vi "read station misc config.vi"(8 "error in":errorcluster, 10 "station idx":i32, 11 "configuration file path in":path) -> (0 "error out":errorcluster, 2 "misc station config":T1, 3 "configuration file path out":path)   [LabVIEW 2018]
uses:
  02.Type Def's/misc station config.ctl
  05.UserVI's/Lambda Power/power supply types.ctl
  05.UserVI's/file io/ini/type defs/ini file actions.ctl
  05.UserVI's/file io/ini/type defs/ini entry value.ctl
  05.UserVI's/file io/ini/type defs/ini entry types.ctl
  05.UserVI's/file io/ini/type defs/ini entry.ctl
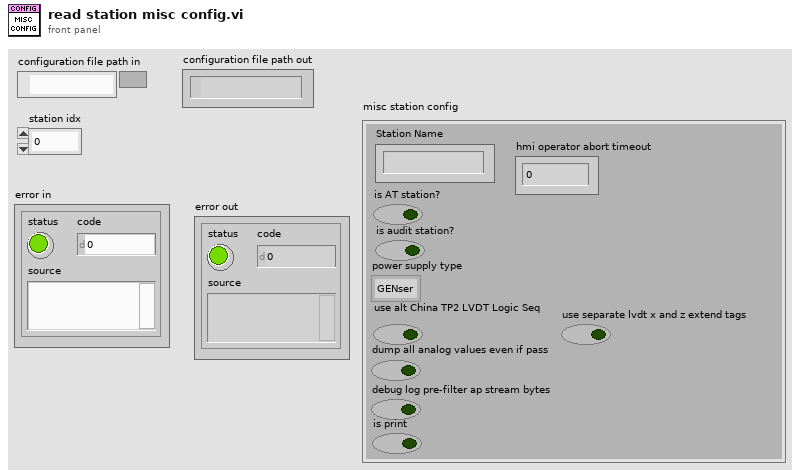
[diagram p1: front panel]
types:
  T1 = typedef "misc station config.ctl" = cluster{"Station Name":string, "is AT station?":bool, "is audit station?":bool, "power supply type":T2, "use alt China TP2 LVDT Logic Seq":bool, "hmi operator abort timeout":u32, "dump all analog values even if pass":bool, "debug log pre-filter ap stream bytes":bool, "use separate lvdt x and z extend tags":bool, "is print":bool}
  T2 = typedef "power supply types.ctl" = enum16{"GENser", "ZUPser", "GENeth", "Manual", "ITECH"}
  T3 = typedef "ini entry value.ctl" = cluster{"Boolean":bool, "Dbl":dbl, "I32":i32, "Path":path, "String":string, "U32":u32}
  T4 = typedef "ini file actions.ctl" = enum16{"read ini", "write ini"}
  T5 = typedef "ini entry.ctl" = cluster{"section":string, "key":string, "type":T6, "default value":T3}
  T6 = typedef "ini entry types.ctl" = enum16{"Boolean", "Double", "I32", "Path", "String", "U32"}
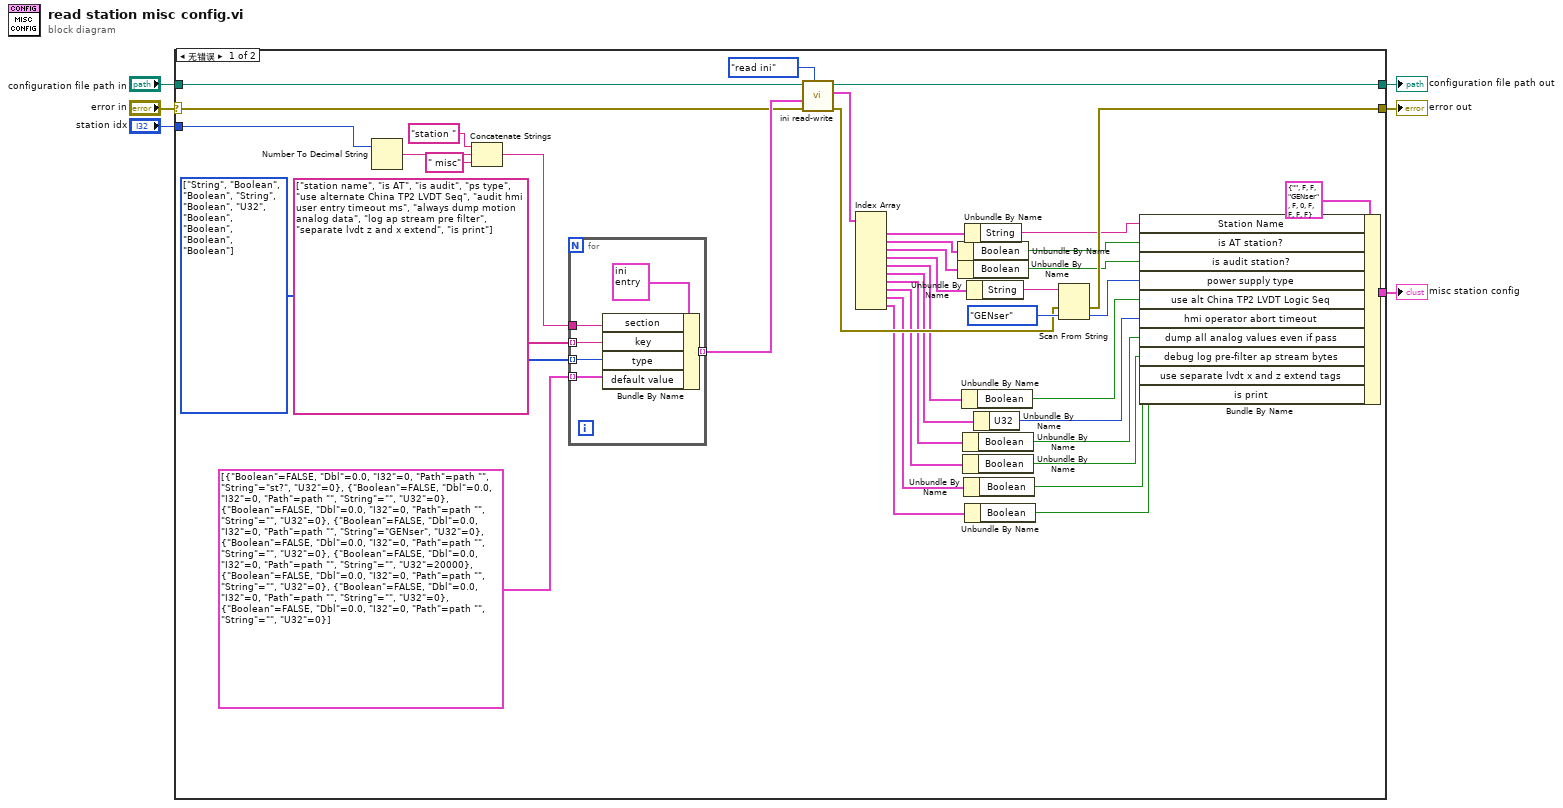
[diagram p0: block diagram]
diagram:
  n1 = case shown="无错误" "error in" {
    selector: "error in" -> [w31 w54]
    tunnel: "configuration file path in" -> [w46 w53]
    tunnel: [w41 w53] -> w5
    tunnel: [w26 w54] -> w4
    tunnel: "station idx" -> [w39 _]
    tunnel: [w18 _] -> w1
    frame No Error {
      w34 = T6[] [enum."String", enum."Boolean", enum."Boolean", enum."String", enum."Boolean", enum."U32", enum."Boolean", enum."Boolean", enum."Boolean", enum."Boolean"] items=["Boolean", "Double", "I32", "Path", "String", "U32"]
      n2 = Number To Decimal String(number=w39) -> (decimal integer string=w38:string)  [unwired: 1 in]
      n3 = Concatenate Strings("station ", w38, " misc" ("string")) -> (w37:string)
      n4 = for {
        tunnel: w37 -> [w51]
        tunnel: string[] ["station name", "is AT", "is audit", "ps type", "use alternate China TP2 LVDT Seq", "audit hmi user entry timeout ms", "always dump motion analog data", "log ap stream pre filter", "separate lvdt z and x extend", "is print"] -> [w50] mode=indexing
        tunnel: w34 -> [w49] mode=indexing
        tunnel: T3[] [{"Boolean"=FALSE, "Dbl"=0.0, "I32"=0, "Path"=path "", "String"="st?", "U32"=0}, {"Boolean"=FALSE, "Dbl"=0.0, "I32"=0, "Path"=path "", "String"="", "U32"=0}, {"Boolean"=FALSE, "Dbl"=0.0, "I32"=0, "Path"=path "", "String"="", "U32"=0}, {"Boolean"=FALSE, "Dbl"=0.0, "I32"=0, "Path"=path "", "String"="GENser", "U32"=0}, {"Boolean"=FALSE, "Dbl"=0.0, "I32"=0, "Path"=path "", "String"="", "U32"=0}, {"Boolean"=FALSE, "Dbl"=0.0, "I32"=0, "Path"=path "", "String"="", "U32"=20000}, {"Boolean"=FALSE, "Dbl"=0.0, "I32"=0, "Path"=path "", "String"="", "U32"=0}, {"Boolean"=FALSE, "Dbl"=0.0, "I32"=0, "Path"=path "", "String"="", "U32"=0}, {"Boolean"=FALSE, "Dbl"=0.0, "I32"=0, "Path"=path "", "String"="", "U32"=0}] -> [w48] mode=indexing
        tunnel: [w47] -> w32 mode=indexing
        n5 = Bundle By Name(cluster=T5 {"section"="", "key"="", "type"=enum."Boolean", "default value"={"Boolean"=FALSE, "Dbl"=0.0, "I32"=0, "Path"=path "", "String"="", "U32"=0}}, "section"=w51, "key"=w50, "type"=w49, "default value"=w48) -> (w47:T5)
      }
      n6 = call "ini read-write.vi"("action"=ini_file_actions."read ini", "error in (no error)"=w31, "ini entry descriptors"=w32, "configuration file path"=w46) -> ("error out"=w25:errorcluster, "values out"=w44:T3[], "configuration file path out"=w41:path)  [unwired: 5 in]
      n7 = Index Array(array=w44) -> (element #1=w43:T3, element #2=w42:T3, element #3=w36:T3, element #4=w29:T3, element #5=w13:T3, element #6=w12:T3, element #7=w11:T3, element #8=w10:T3, element #9=w9:T3, element #10=w8:T3)  [unwired: 10 in]
      n8 = Unbundle By Name(w42) -> ("Boolean"=w22:bool)
      n9 = Unbundle By Name(w36) -> ("Boolean"=w21:bool)
      n10 = Unbundle By Name(w13) -> ("Boolean"=w19:bool)
      n11 = Unbundle By Name(w11) -> ("Boolean"=w16:bool)
      n12 = Unbundle By Name(w10) -> ("Boolean"=w15:bool)
      n13 = Unbundle By Name(w9) -> ("Boolean"=w14:bool)
      n14 = Unbundle By Name(w43) -> ("String"=w23:string)
      n15 = Unbundle By Name(w8) -> ("Boolean"=w7:bool)
      n16 = Unbundle By Name(w29) -> ("String"=w27:string)
      n17 = Unbundle By Name(w12) -> ("U32"=w17:u32)
      n18 = Scan From String(input string=w27, error in=w25, default 1=power_supply_types."GENser" ("power supply model")) -> (error out=w26:errorcluster, output 1=w20:T2)  [unwired: 2 in, 2 out]
      n19 = Bundle By Name(cluster=T1 {"Station Name"="", "is AT station?"=FALSE, "is audit station?"=FALSE, "power supply type"=enum."GENser", "use alt China TP2 LVDT Logic Seq"=FALSE, "hmi operator abort timeout"=0, "dump all analog values even if pass"=FALSE, "debug log pre-filter ap stream bytes"=FALSE, "use separate lvdt x and z extend tags"=FALSE, "is print"=FALSE} ("misc station config"), "Station Name"=w23, "is AT station?"=w22, "is audit station?"=w21, "power supply type"=w20, "use alt China TP2 LVDT Logic Seq"=w19, "hmi operator abort timeout"=w17, "dump all analog values even if pass"=w16, "debug log pre-filter ap stream bytes"=w15, "use separate lvdt x and z extend tags"=w14, "is print"=w7) -> (w18:T1)
    }
    frame Error {
    }
  }
  "configuration file path out" <- w5
  "error out" <- w4
  "misc station config" <- w1
